vi "CreateUserEvents.vi"(8 "error in (no error)":errorcluster, 11 "UserEvents":T1) -> (0 "error out":errorcluster, 3 "UserEvents out":T1)   [LabVIEW 2022 SP3, in "GIS Printer.lvclass"]
uses:
  GIS Printer.lvclass
  Typedefs/UserEvents.ctl
  Typedefs/API Event Data.ctl
  Typedefs/API Task State.ctl
  Typedefs/Status Cluster.ctl
  Typedefs/AbortEventData--Cluster.ctl
  Typedefs/GIS Status--Cluster.ctl
  Typedefs/HeadEnableStatus--cluster.ctl
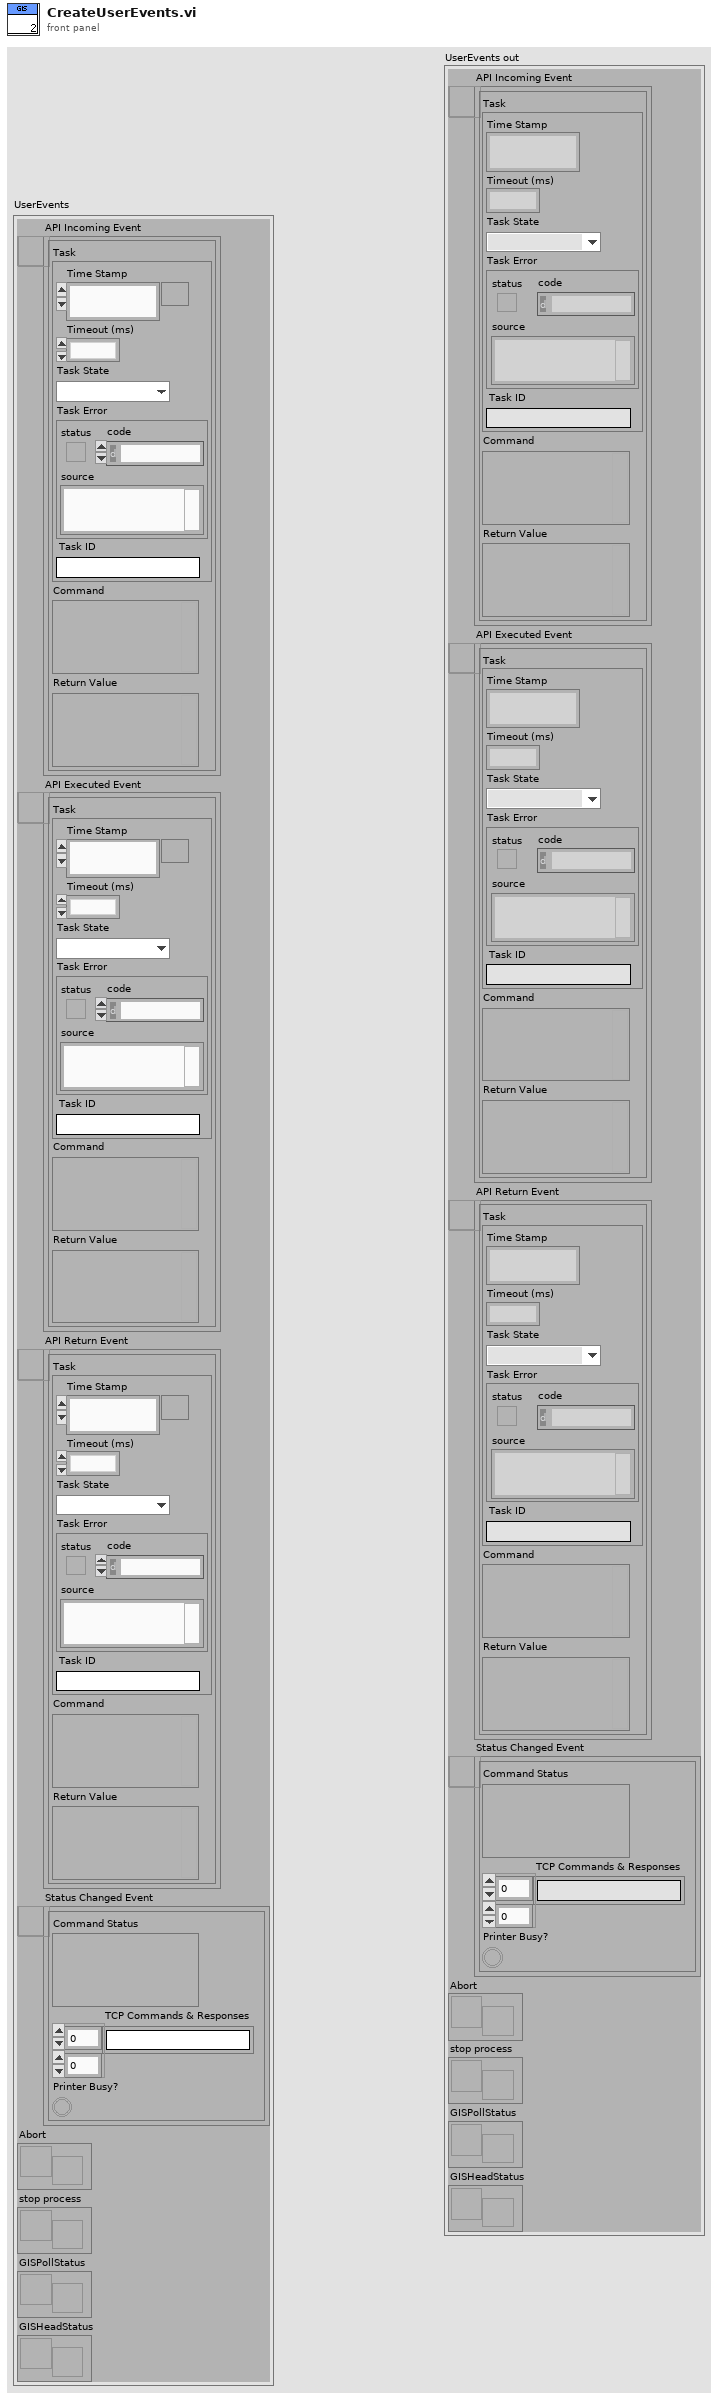
[diagram p1: front panel]
types:
  T1 = typedef "GIS Printer.lvclass/UserEvents.ctl" = cluster{"API Incoming Event":refnum<user-event>, "API Executed Event":refnum<user-event>, "API Return Event":refnum<user-event>, "Status Changed Event":refnum<user-event>, "Abort":refnum<user-event>, "stop process":refnum<user-event>, "GISPollStatus":refnum<user-event>, "GISHeadStatus":refnum<user-event>}
  T2 = typedef "HeadEnableStatus--cluster.ctl" = cluster{"PH1_Enable":bool, "PH2_Enable":bool, "PH3_Enable":bool, "PH4_Enable":bool, "PH5_Enable":bool, "PH6_Enable":bool}
  T3 = typedef "GIS Status--Cluster.ctl" = cluster{"HeadEnabled":bool, "SpitEnabled":bool, "HeaterEnabled":bool, "TargetTemperature":dbl, "CurrentTemperature":dbl}
  T4 = typedef "GIS Printer.lvclass/Status Cluster.ctl" = cluster{"Command Status":variant, "TCP Commands & Responses":string[][], "Printer Busy?":bool}
  T5 = typedef "GIS Printer.lvclass/API Event Data.ctl" = cluster{"Task":cluster{"Time Stamp":timestamp, "Timeout (ms)":u32, "Task State":T6, "Task Error":errorcluster, "Task ID":string}, "Command":variant, "Return Value":variant}
  T6 = typedef "GIS Printer.lvclass/API Task State.ctl" = enum16{"Completed", "Errored", "Pending"}
  T7 = typedef "AbortEventData--Cluster.ctl" = cluster{"Abort":bool}
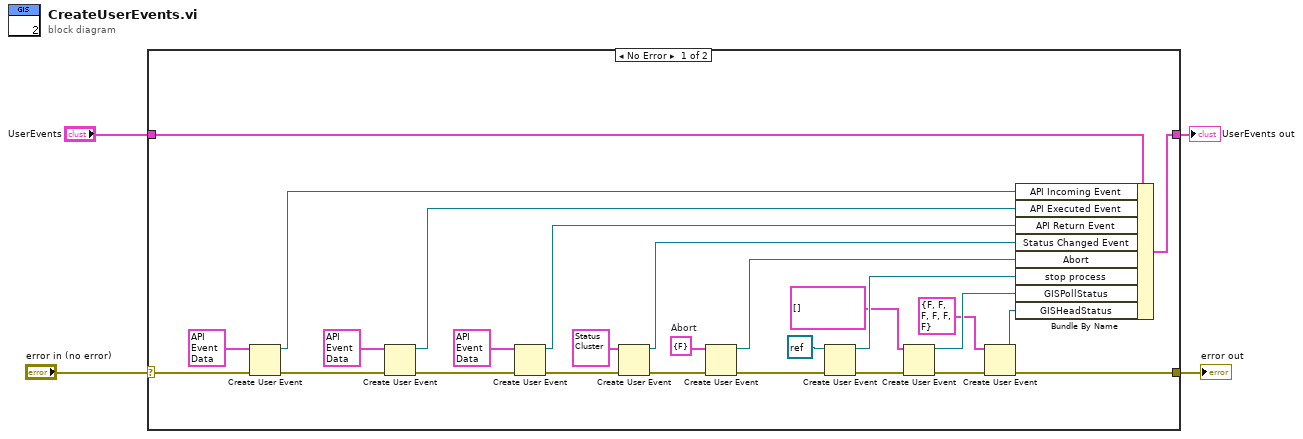
[diagram p0: block diagram]
diagram:
  n1 = case shown="No Error" "error in (no error)" {
    selector: "error in (no error)" -> [w27 w33]
    tunnel: [w6 w33] -> w3
    tunnel: "UserEvents" -> [w31 w32]
    tunnel: [w30 w32] -> w1
    frame No Error {
      w17 = T7 {"Abort"=FALSE}  # Abort
      n2 = Create User Event(user event datatype=T5 {"Task"={"Time Stamp"=timestamp(0 s since 1904-01-01), "Timeout (ms)"=0, "Task State"=enum."Completed", "Task Error"={"status"=FALSE, "code"=0, "source"=""}, "Task ID"=""}, "Command"=variant(enum16{"Event 1"} enum."Event 1"), "Return Value"=variant(string "")} ("API Event Data"), error in=w27) -> (user event=w28:refnum<user-event>, error out=w25:errorcluster)
      n3 = Create User Event(user event datatype=T5 {"Task"={"Time Stamp"=timestamp(0 s since 1904-01-01), "Timeout (ms)"=0, "Task State"=enum."Completed", "Task Error"={"status"=FALSE, "code"=0, "source"=""}, "Task ID"=""}, "Command"=variant(enum16{"Event 1"} enum."Event 1"), "Return Value"=variant(string "")} ("API Event Data"), error in=w25) -> (user event=w24:refnum<user-event>, error out=w22:errorcluster)
      n4 = Create User Event(user event datatype=T5 {"Task"={"Time Stamp"=timestamp(0 s since 1904-01-01), "Timeout (ms)"=0, "Task State"=enum."Completed", "Task Error"={"status"=FALSE, "code"=0, "source"=""}, "Task ID"=""}, "Command"=variant(enum16{"Event 1"} enum."Event 1"), "Return Value"=variant(string "")} ("API Event Data"), error in=w22) -> (user event=w21:refnum<user-event>, error out=w19:errorcluster)
      n5 = Create User Event(user event datatype=T4 {"Command Status"=variant, "TCP Commands & Responses"=[], "Printer Busy?"=FALSE} ("Status"), error in=w19) -> (user event=w18:refnum<user-event>, error out=w16:errorcluster)
      n6 = Create User Event(user event datatype=w17, error in=w16) -> (user event=w15:refnum<user-event>, error out=w13:errorcluster)
      n7 = Create User Event(user event datatype=refnum<notifier> refnum ("notifier out"), error in=w13) -> (user event=w12:refnum<user-event>, error out=w11:errorcluster)
      n8 = Create User Event(user event datatype=T3[] [] ("GISHeadStatus"), error in=w11) -> (user event=w9:refnum<user-event>, error out=w7:errorcluster)
      n9 = Create User Event(user event datatype=T2 {"PH1_Enable"=FALSE, "PH2_Enable"=FALSE, "PH3_Enable"=FALSE, "PH4_Enable"=FALSE, "PH5_Enable"=FALSE, "PH6_Enable"=FALSE} ("HeadStatus"), error in=w7) -> (user event=w5:refnum<user-event>, error out=w6:errorcluster)
      n10 = Bundle By Name(cluster=w31, "API Incoming Event"=w28, "API Executed Event"=w24, "API Return Event"=w21, "Status Changed Event"=w18, "Abort"=w15, "stop process"=w12, "GISPollStatus"=w9, "GISHeadStatus"=w5) -> (w30:T1)
    }
    frame Error {
    }
  }
  "error out" <- w3
  "UserEvents out" <- w1
